vi "Set Controls Disable (selective).vi"(8 "error in (no error)":errorcluster, 10 "disabled":T1(ring), 11 "ctrls":refnum<vi>[](array[refnum])) -> (0 "error out":errorcluster, 3 "ctrls dup":refnum<vi>[](array[refnum]))   [LabVIEW 2017]
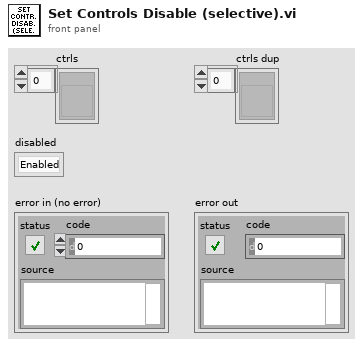
[diagram p1: front panel]
types:
  T1 = enum8{"Enabled", "Disabled", "Disabled and Grayed Out"}
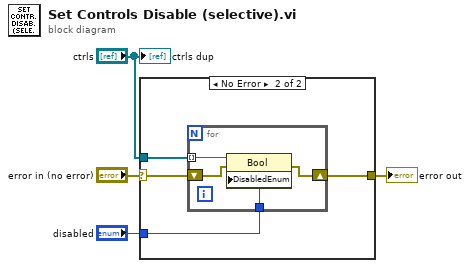
[diagram p0: block diagram]
diagram:
  n1 = case shown="No Error" "error in (no error)" {
    selector: "error in (no error)" -> [w5 w6]
    tunnel: "disabled" -> [_ w9]
    tunnel: "ctrls" -> [_ w8]
    tunnel: [w5 w7] -> w2
    frame Error {
    }
    frame No Error {
      n2 = for {
        tunnel: w8 -> [w13] mode=indexing
        tunnel: w9 -> [w12]
        shift-right: [w10] -> w7
        shift-left: w6 -> [w11]
        n3 = property on="Property Node" class="Bool"(reference=w13, error in=w11, "DisabledEnum"=w12) -> (error out=w10:errorcluster)  [unwired: 1 out]
      }
    }
  }
  "error out" <- w2
  "ctrls dup" <- "ctrls"
